vi "Get Parent.vi"(8 "Error In":errorcluster, 11 "reference in":refnum<class "OD Sub-Entry.lvclass">) -> (0 "Error Out":errorcluster, 2 "Parent":refnum<class "OD Entry.lvclass">, 3 "reference out":refnum<class "OD Sub-Entry.lvclass">)   [LabVIEW 2019, in "Electronic Datasheet.lvlib" / "OD Sub-Entry.lvclass"]
uses:
  OD Sub-Entry.lvclass
  OD Entry/OD Entry.lvclass
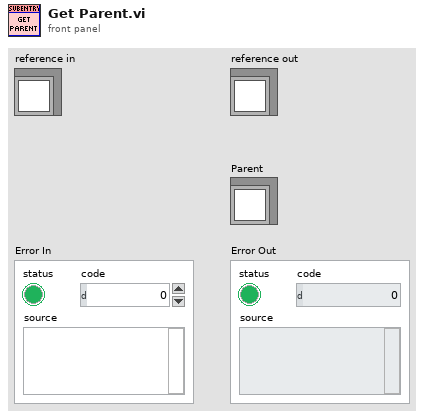
[diagram p1: front panel]
types:
  T1 = typedef "Electronic Datasheet.lvlib/OD Sub-Entry.lvclass/ObjectAttributes.ctl" = cluster{"Parent":refnum<class "OD Entry.lvclass">}
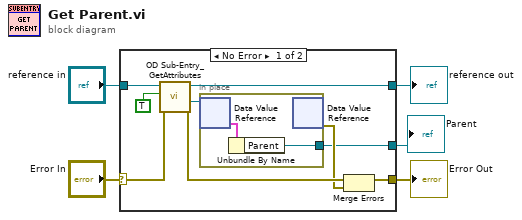
[diagram p0: block diagram]
diagram:
  n1 = case shown="No Error" "Error In" {
    selector: "Error In" -> [w14 w18]
    tunnel: [w12 w18] -> w4
    tunnel: [w9 w17] -> w2
    tunnel: "reference in" -> [w10 w17]
    tunnel: [w6 _] -> w1
    frame No Error {
      n2 = call "OD Sub-Entry_GetAttributes.vi"("Error In"=w14, "OnlyGetDvrReference(False)"=TRUE, "reference in"=w10) -> ("Error Out"=w13:errorcluster, "DataRef"=w8:refnum<data-value>, "reference out"=w9:refnum<class "OD Sub-Entry.lvclass">)  [unwired: 5 in, 1 out]
      n3 = in-place {
        in-place-border: [w16] -> w6
        n4 = in-place-dvr #1(w8) -> (w15:T1)  [unwired: 1 out]
        n5 = Unbundle By Name(w15) -> ("Parent"=w16:refnum<class "OD Entry.lvclass">)
        n6 = in-place-dvr #1() -> (w11:errorcluster)  [unwired: 1 in, 1 out]
      }
      n7 = Merge Errors(w13, w11) -> (w12:errorcluster)
    }
    frame Error {
    }
  }
  "Error Out" <- w4
  "reference out" <- w2
  "Parent" <- w1
